vi "UDP ROS Reciever.vi"(8 "error in (no error)":errorcluster, 9 "ENQUE DIRECTLY":refnum<queue>, 10 "milliseconds to wait":u32, 11 "UDP Network Connection in":refnum<k16>) -> (0 "error out":errorcluster)   [LabVIEW 2016]
uses:
  Globale Variablen VI/AutonomousMode.vi
  Globale Variablen VI/Global Variables.vi
  Globale Variablen VI/RadSensoren.vi
  Globale Variable/Globale Variable.vi
panel:
  out "data out":string
  out "vs recieved":dbl
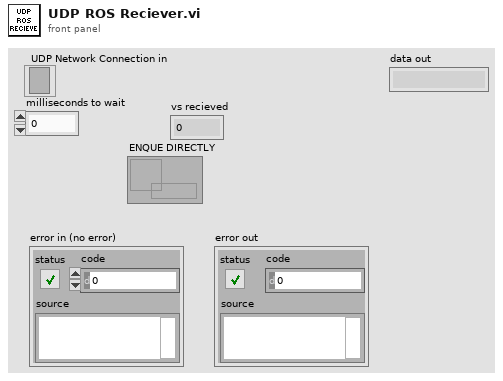
[diagram p1: front panel]
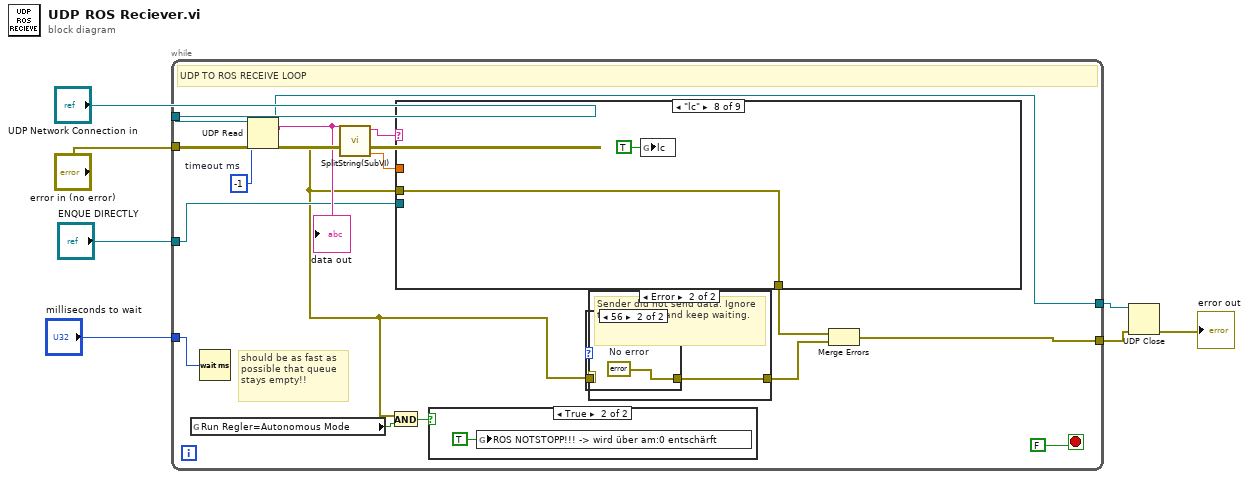
[diagram p0: block diagram]
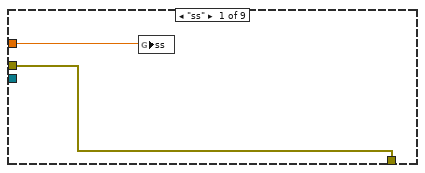
[diagram p3: hidden frame]
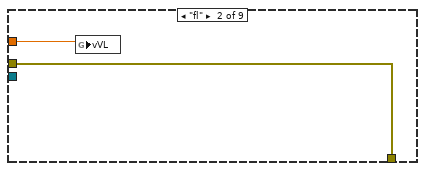
[diagram p4: hidden frame]
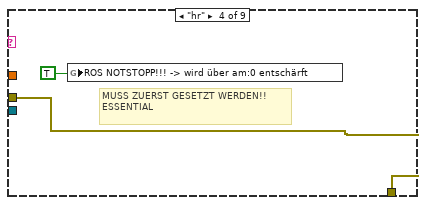
[diagram p6: hidden frame]
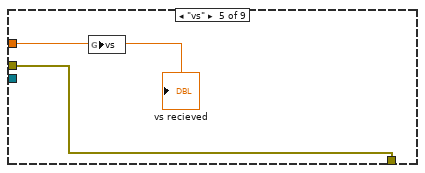
[diagram p7: hidden frame]
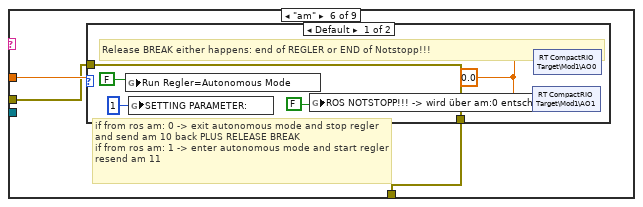
[diagram p8: hidden frame]
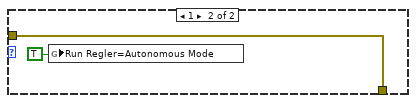
[diagram p9: hidden frame]
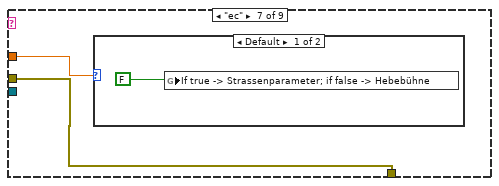
[diagram p10: hidden frame]
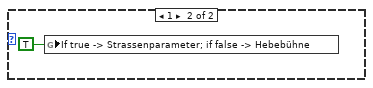
[diagram p11: hidden frame]
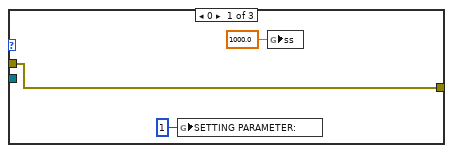
[diagram p13: hidden frame]
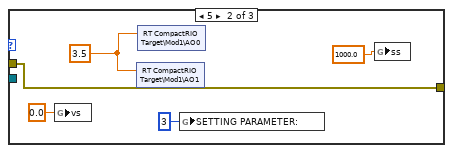
[diagram p14: hidden frame]
diagram:
  n1 = while {
    tunnel: [w20] -> w6
    tunnel: "UDP Network Connection in" -> [w22]
    tunnel: "error in (no error)" -> [w21]
    tunnel: "milliseconds to wait" -> [w16]
    tunnel: [w13] -> w2
    tunnel: "ENQUE DIRECTLY" -> [w12]
    stop <- FALSE stop-if-true
    w23 = -1  # timeout ms
    # "should be as fast as possible that queue stays empty!!"
    # "UDP TO ROS RECEIVE LOOP"
    n2 = global read "AutonomousMode.vi" "Run Regler=Autonomous Mode"() -> (w10:bool)
    n3 = Wait (ms)(milliseconds to wait=w16) -> ()  [unwired: 1 out]
    n4 = UDP Read(connection ID=w22, timeout ms (25000)=w23, 8:w21) -> (data out=w17:string, error out=w9:errorcluster, 3:w20:refnum<k16>)  [unwired: 3 out]
    "data out" <- w17
    n5 = call "SplitString(SubVI).vi"("data in"=w17) -> ("Numeric"=w19:dbl, "String 3"=w18:string)  [unwired: 9 in]
    n6 = And(x=w9, y=w10) -> (x .and. y?=w11:bool)
    n7 = case shown="\"lc\"" w18 {
      tunnel: w19 -> [w26 w28 _ _ w33 w36 w45 _ w53]
      tunnel: w9 -> [w25 w27 w29 w31 w32 w35 w44 w49 w52]
      tunnel: [w25 w27 w29 w31 w32 w34 w44 w49 w51] -> w14
      tunnel: w12 -> [_ _ _ _ _ _ _ _ w50]
      frame "ss" {
        n8 = global write "Global Variables.vi" "ss"(w26) -> ()
      }
      frame "fl" {
        n9 = global write "RadSensoren.vi" "vVL"(w28) -> ()
      }
      frame Default {
      }
      frame "hr" {
        # "MUSS ZUERST GESETZT WERDEN!! ESSENTIAL"
        n10 = global write "AutonomousMode.vi" "ROS NOTSTOPP!!! -> wird über am:0 entschärft"(TRUE ("Run Regler=Autonomous Mode")) -> ()
      }
      frame "vs" {
        n11 = global write "RadSensoren.vi" "vs"(w33) -> ()
        "vs recieved" <- w33
      }
      frame "am" {
        # "if from ros am: 0 -> exit autonomous mode and stop regler and send am 10 back PLUS RELEASE BREAK\nif from ros am: 1 -> enter autonomous mode and start regler resend am 11"
        n12 = case shown="Default" w36 {
          tunnel: w35 -> [w38 w42]
          tunnel: [w38 w42] -> w34
          frame Default {
            w37 = 0.0
            # "Release BREAK either happens: end of REGLER or END of Notstopp!!!"
            n13 = global write "AutonomousMode.vi" "Run Regler=Autonomous Mode"(FALSE ("Run Regler=Autonomous Mode")) -> ()
            n14 = global write "Global Variables.vi" "SETTING PARAMETER:"(1 ("SETTING PARAMETER:")) -> ()
            n15 = global write "AutonomousMode.vi" "ROS NOTSTOPP!!! -> wird über am:0 entschärft"(FALSE ("Run Regler=Autonomous Mode")) -> ()
            n16 = shared-variable "RT CompactRIO Target\\Mod1\\AO1"(w37) -> ()  [unwired: 1 in, 1 out]
            n17 = shared-variable "RT CompactRIO Target\\Mod1\\AO0"(w37) -> ()  [unwired: 1 in, 1 out]
          }
          frame 1 {
            n18 = global write "AutonomousMode.vi" "Run Regler=Autonomous Mode"(TRUE) -> ()
          }
        }
      }
      frame "ec" {
        n19 = case shown="Default" w45 {
          frame Default {
            n20 = global write "AutonomousMode.vi" "If true -> Strassenparameter; if false -> Hebebühne"(FALSE) -> ()
          }
          frame 1 {
            n21 = global write "AutonomousMode.vi" "If true -> Strassenparameter; if false -> Hebebühne"(TRUE) -> ()
          }
        }
      }
      frame "lc" {
        n22 = global write "Globale Variable.vi" "lc"(TRUE ("lc")) -> ()
      }
      frame "cc" {
        n23 = case shown="Default" w53 {
          tunnel: w52 -> [w54 w59 w62]
          tunnel: [w54 w59 w62] -> w51
          tunnel: w50 -> [_ _ _]
          frame 0 {
            n24 = global write "Global Variables.vi" "SETTING PARAMETER:"(1 ("SETTING PARAMETER:")) -> ()
            n25 = global write "Global Variables.vi" "ss"(1000.0 ("ss")) -> ()
          }
          frame 5 {
            w58 = 3.5
            n26 = global write "RadSensoren.vi" "vs"(0.0 ("vs")) -> ()
            n27 = shared-variable "RT CompactRIO Target\\Mod1\\AO1"(w58) -> ()  [unwired: 1 in, 1 out]
            n28 = shared-variable "RT CompactRIO Target\\Mod1\\AO0"(w58) -> ()  [unwired: 1 in, 1 out]
            n29 = global write "Global Variables.vi" "SETTING PARAMETER:"(3 ("SETTING PARAMETER:")) -> ()
            n30 = global write "Global Variables.vi" "ss"(1000.0 ("ss")) -> ()
          }
          frame Default {
          }
        }
      }
    }
    n31 = case shown="True" w11 {
      frame False {
      }
      frame True {
        n32 = global write "AutonomousMode.vi" "ROS NOTSTOPP!!! -> wird über am:0 entschärft"(TRUE ("ROS NOTSTOPP!!! -> wird über am:0 entschärft")) -> ()
      }
    }
    n33 = case shown="Error" w9 {
      selector: w9 -> [w63 w65]
      tunnel: [w63 w64] -> w15
      frame No Error {
        # "Sender sent data. Update the chart value."
      }
      frame Error {
        # "Sender did not send data. Ignore timeout error and keep waiting."
        n34 = Unbundle By Name(w65) -> ("code"=w66:i32)
        n35 = case shown="56" w66 {
          tunnel: w65 -> [w67 _]
          tunnel: [w67 w68] -> w64
          frame Default {
          }
          frame 56 {
            w68 = errorcluster {"status"=FALSE, "code"=0, "source"=""}  # No error
          }
        }
      }
    }
    n36 = Merge Errors(w14, w15) -> (w13:errorcluster)
  }
  n37 = UDP Close(connection ID=w6, 8:w2) -> (error out=→"error out":errorcluster)  [unwired: 1 out]
